vi "MK_Steps per second to Velocity.vi"(11 "Steps/sec (3-365)":dbl) -> (3 "Velocity":string)   [LabVIEW 2014]
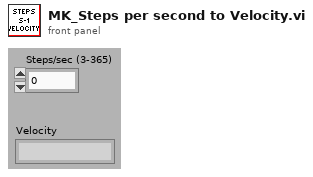
[diagram p1: front panel]
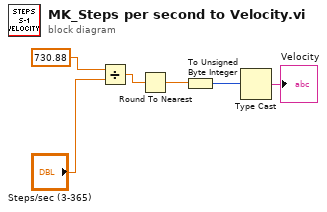
[diagram p0: block diagram]
diagram:
  n1 = Divide(x=730.88, y="Steps/sec (3-365)") -> (x/y=w5:dbl)
  n2 = Round To Nearest(number=w5) -> (nearest integer value=w4:dbl)
  n3 = To Unsigned Byte Integer(number=w4) -> (unsigned 8bit integer=w2:u8)
  n4 = Type Cast(x=w2) -> (*(type *) &x=→"Velocity":string)  [unwired: 1 in]
